vi "Unmarshal.vi"(8 "error in (no error)":errorcluster, 10 "Buffer":u8[](array[numeric]), 11 "int32 in":refnum<class "bool.lvclass">) -> (0 "error out":errorcluster, 2 "Buffer Count":i32=8, 3 "int32 out":refnum<class "bool.lvclass">)   [LabVIEW 2020, in "Protobuf RAW.lvlib" / "bool.lvclass"]
uses:
  bool.lvclass
  bool.lvclass/bool.ctl
  Protobuf RAW.lvlib
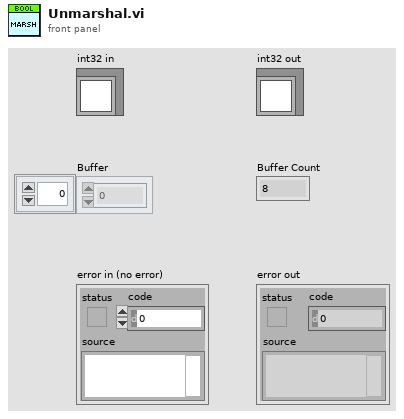
[diagram p1: front panel]
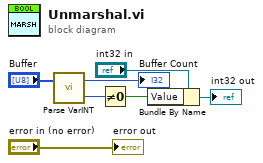
[diagram p0: block diagram]
diagram:
  n1 = call "Parse VarINT.vi"("Buffer"="Buffer") -> ("Numeric"=w3:u64, "Bytes"=→"Buffer Count":i32)  [unwired: 1 in]
  n2 = Not Equal To 0?(x=w3) -> (x != 0?=w2:bool)
  n3 = Bundle By Name(cluster="int32 in", "Value"=w2) -> (→"int32 out":refnum<class "bool.lvclass">)
  "error out" <- "error in (no error)"
